vi "Configure Measurement (Occupied Bandwidth).vi"(0 "VISA resource name":refnum<visa-resource-name>, 1 "Enable Max Hold (F: Disable)":bool, 5 "Enable Limit Test (F: Disable)":bool, 7 "Occupied Bandwidth Percent Power (99 %)":dbl=99.0, 9 "X dB (-26 dB)":dbl=-26.0, 11 "error in (no error)":errorcluster, 12 "Bandwidth Filter Type (0: Gaussian)":i32(ring) items=["Gaussian", "Flattop"], 13 "Limit Checking Frequency (5E+6 Hz)":dbl=5000000.0) -> (4 "VISA resource name out":refnum<visa-resource-name>, 15 "error out":errorcluster)   [LabVIEW 2018, in "Agilent MXA Series.lvlib"]
doc: "Sets the Occupied Bandwidth measurement parameters."
uses:
  Agilent MXA Series.lvlib
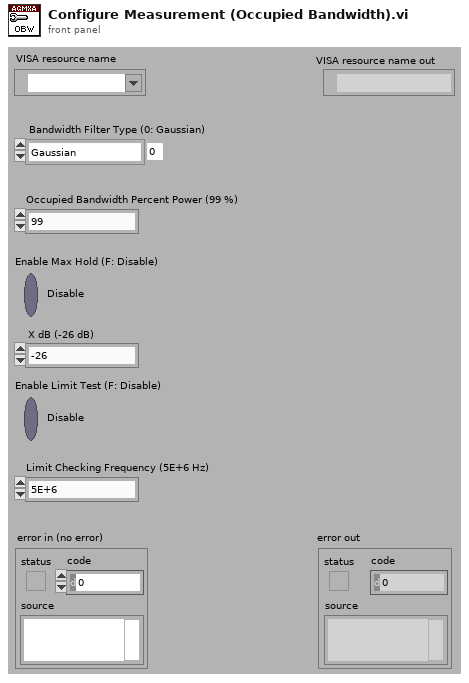
[diagram p1: front panel]
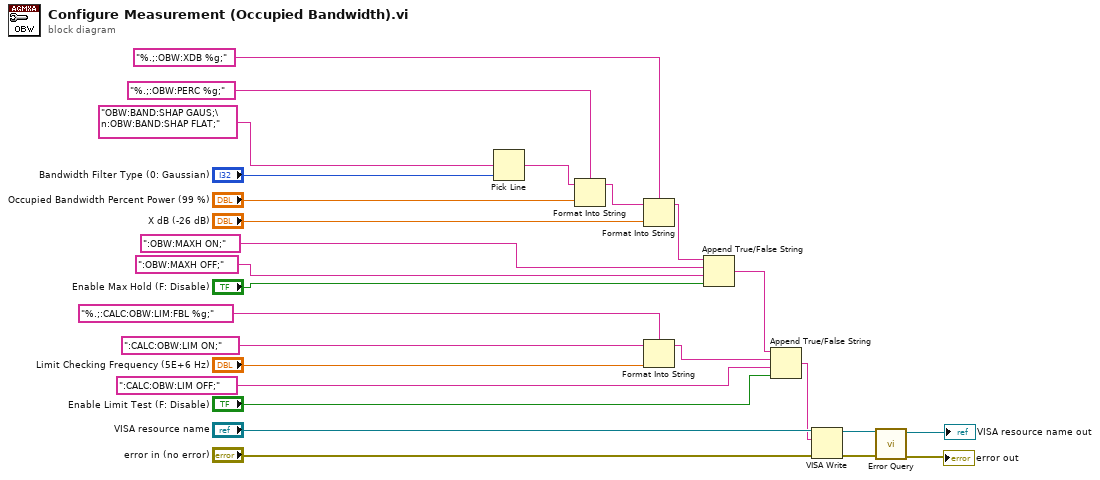
[diagram p0: block diagram]
diagram:
  n1 = Pick Line(multi-line string="OBW:BAND:SHAP GAUS;\n:OBW:BAND:SHAP FLAT;", line index="Bandwidth Filter Type (0: Gaussian)") -> (output string=w4:string)  [unwired: 1 in]
  n2 = Format Into String(format string="%.;:OBW:PERC %g;", initial string=w4, "Occupied Bandwidth Percent Power (99 %)") -> (resulting string=w5:string)  [unwired: 1 in, 1 out]
  n3 = Format Into String(format string="%.;:OBW:XDB %g;", initial string=w5, "X dB (-26 dB)") -> (resulting string=w3:string)  [unwired: 1 in, 1 out]
  n4 = Format Into String(format string="%.;:CALC:OBW:LIM:FBL %g;", initial string=":CALC:OBW:LIM ON;", "Limit Checking Frequency (5E+6 Hz)") -> (resulting string=w13:string)  [unwired: 1 in, 1 out]
  n5 = Append True/False String(1:"Enable Max Hold (F: Disable)", 2:":OBW:MAXH OFF;" ("false string"), 3:":OBW:MAXH ON;" ("true string"), 4:w3) -> (0:w2:string)
  n6 = Append True/False String(1:"Enable Limit Test (F: Disable)", 2:":CALC:OBW:LIM OFF;" ("false string"), 3:w13, 4:w2) -> (0:w1:string)
  n7 = VISA Write(VISA resource name="VISA resource name", write buffer=w1, error in (no error)="error in (no error)") -> (VISA resource name out=w8:refnum<visa-resource-name>, error out=w9:errorcluster)  [unwired: 1 out]
  n8 = call "Error Query.vi"("error in (no error)"=w9, "VISA resource name"=w8) -> ("error out"=→"error out":errorcluster, "VISA resource name out"=→"VISA resource name out":refnum<visa-resource-name>)  [unwired: 6 in, 2 out]
